vi "Oxford-VRM-Main-Launcher.vi"() -> ()   [LabVIEW 2019]
doc: "This VI will launch the PPMS 2 Instrument backend that will contunously monitor the state of the instrument and log to the DSC. The user has the option of launching a user interface (default) or allowing the backend to run headless. Run \"Launch PPMS2 UI.vi\" here or on a different computer to have a remote user interface. You can also use the APIs like \"Get Temperturature\" interact programmatically with the PPMS 2 Instrument backend."
uses:
  <vilib>/JKI/JKI SMO/SMO/Typedefs/SMOState --Enum.ctl
  SMOs/Instrument.OxfordVRM UI/Instrument.OxfordVRM UI.lvclass
  C:/Program Files (x86)/National Instruments/LabVIEW 2019/vi.lib/JKI/JKI SMO/SMO/SMO.lvclass
  C:/Program Files (x86)/National Instruments/LabVIEW 2019/vi.lib/JKI/JKI SMO/SMO.UI/SMO.UI.lvclass
  C:/Program Files (x86)/National Instruments/LabVIEW 2019/user.lib/LevyLab/Instrument Framework/SMOs/Instrument UI/Instrument UI.lvclass
  SMOs/Instrument.OxfordVRM/Instrument.OxfordVRM.lvclass
  C:/Program Files (x86)/National Instruments/LabVIEW 2019/user.lib/LevyLab/Instrument Framework/SMOs/Instrument/Instrument.lvclass
  <vilib>/JKI/JKI SMO/SMO/SMO.lvclass/SMO.ctl
  <vilib>/JKI/JKI SMO/SMO.UI/SMO.UI.lvclass/SMO.UI.ctl
  <vilib>/JKI/JKI SMO/SMO/Private/ReftoDVR--SMO.vi
  <vilib>/JKI/JKI SMO/SMO.UI/SMO.UI.ReftoDVR.vi
  <vilib>/JKI/JKI SMO/SMO/SMO.lvclass
  <vilib>/JKI/JKI SMO/SMO.UI/SMO.UI.lvclass
  <userlib>/LevyLab/Instrument Framework/SMOs/Instrument UI/Instrument UI.lvclass
  <userlib>/LevyLab/Instrument Framework/SMOs/Instrument/Instrument.lvclass
panel:
  out "version":string="v20/10/28"
  in  "Examine Configuration.ini":bool
  in  "Debug Mode":bool
  in  "Stop Application":bool caption="Stop"
  in  "Start Application":bool caption="Play"
  in  "Splash Status":string="Push Start to Start..." caption="String"
  out "UI SMO State":T1=enum."Stopped"
  out "SMO State":T1
  out "error out":errorcluster
  # "OI 1820"
  # "v"
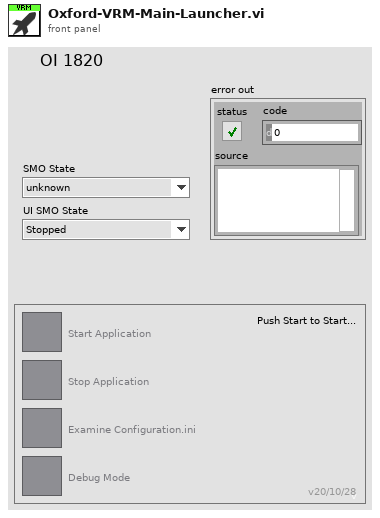
[diagram p1: front panel]
types:
  T1 = typedef "SMO.lvclass/SMOState --Enum.ctl" = enum16{"unknown", "Created", "Started", "Stopped"}
  T2 = enum32{"Invalid", "Standard", "Closed", "Hidden", "Minimized", "Maximized"}
  T3 = enum32{"invalid app kind", "Development System", "Run Time System", "Student Edition", "Embedded LabVIEW", "Evaluation", "Custom"}
  T4 = cluster{"Core":cluster{"Current VI Reference":refnum<vi>, "Close Panel on Exit?":bool}, "Instrument.OxfordVRM":refnum<class "Instrument.OxfordVRM.lvclass">, "Instrument.OxfordVRM UI":refnum<class "Instrument.OxfordVRM UI.lvclass">}
  T5 = cluster{"Current VI Reference":refnum<vi>, "Close Panel on Exit?":bool}
  T6 = typedef "SMO.lvclass/Public Events.ctl" = cluster{"Error":refnum<user-event>, "State":refnum<user-event>, "Reserve State":refnum<user-event>}
  T7 = typedef "SMO.UI.lvclass/PublicEvents--Cluster.ctl" = cluster{"UI Hidden":refnum<user-event>, "UI State":refnum<user-event>}
  T8 = cluster{"Event Registration Refnum":refnum<event-registration>, "Event Registration Refnum":refnum<event-registration>}
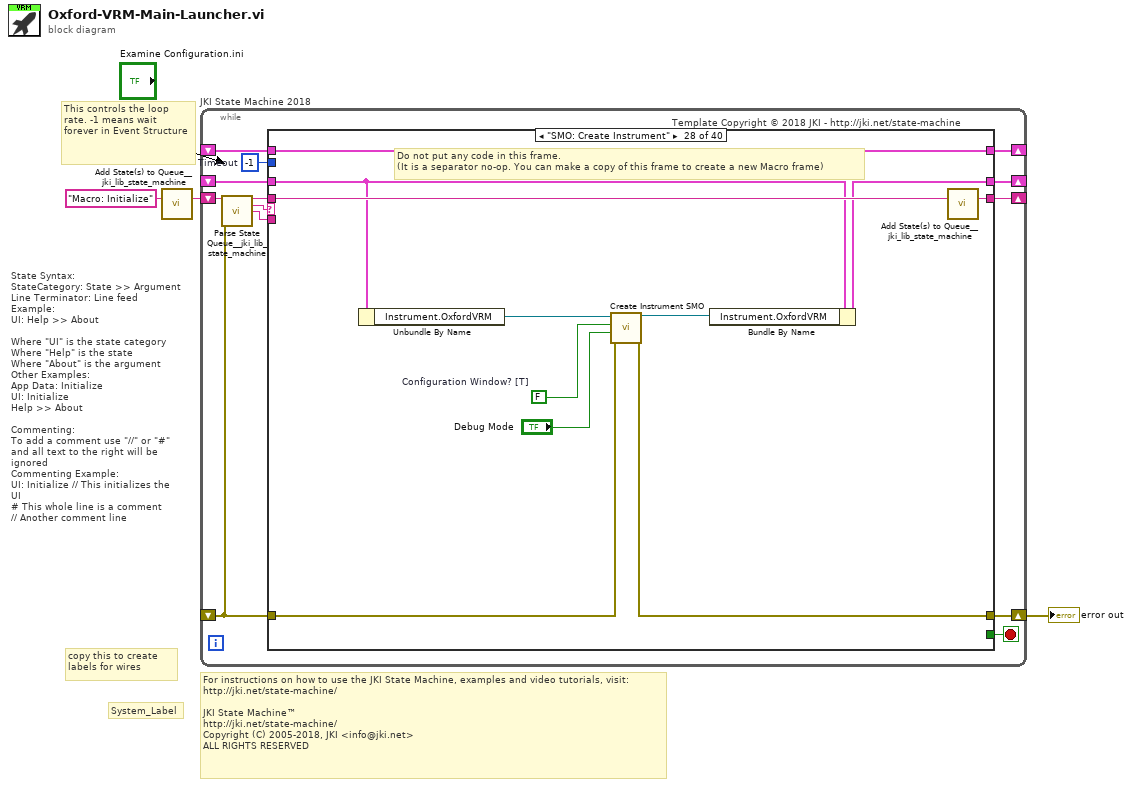
[diagram p0: block diagram]
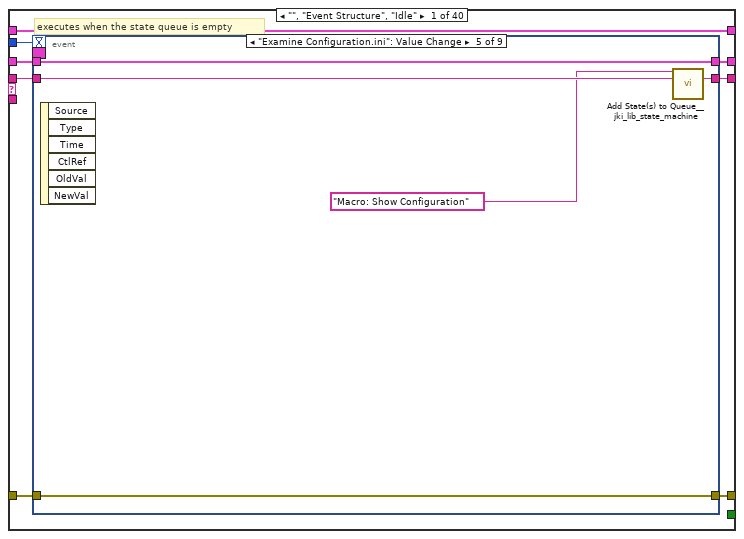
[diagram p2: hidden frame]
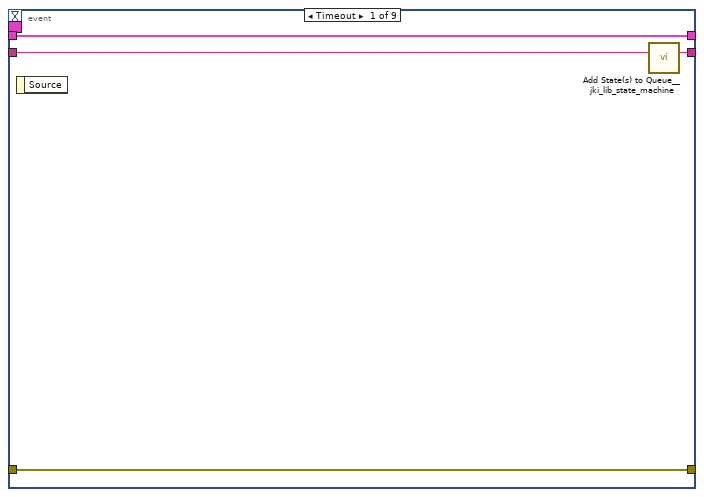
[diagram p3: hidden frame]
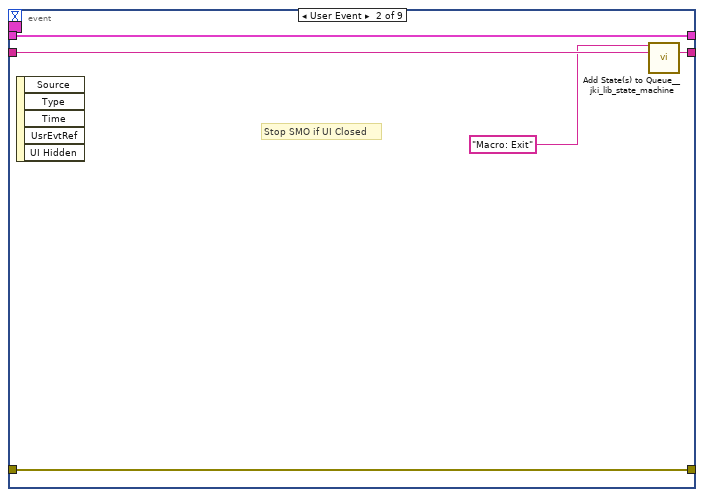
[diagram p4: hidden frame]
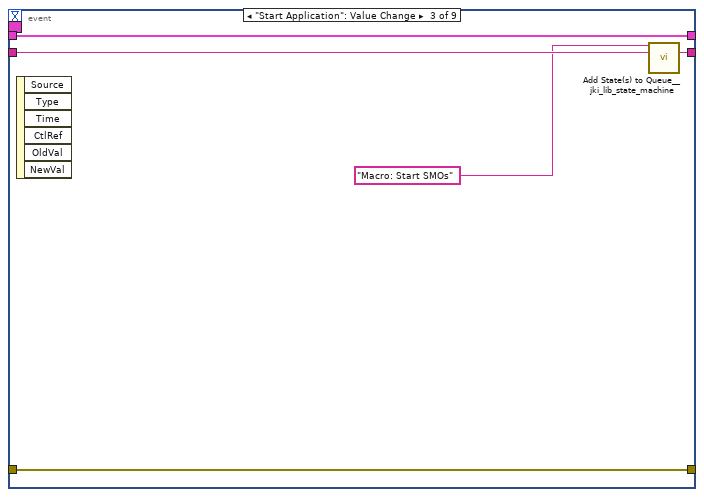
[diagram p5: hidden frame]
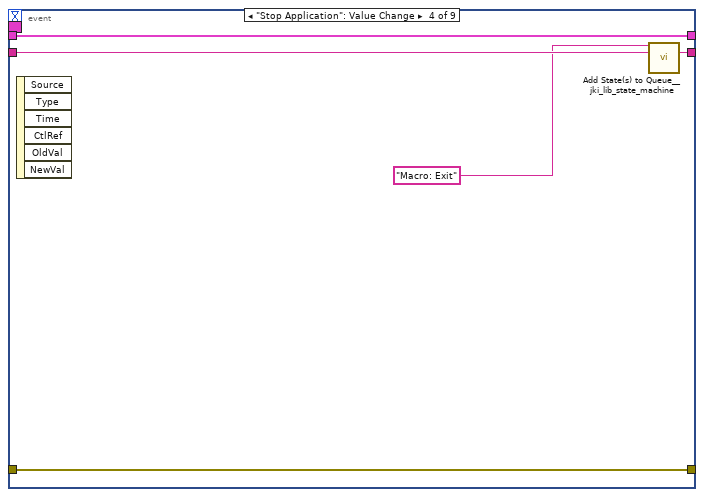
[diagram p6: hidden frame]
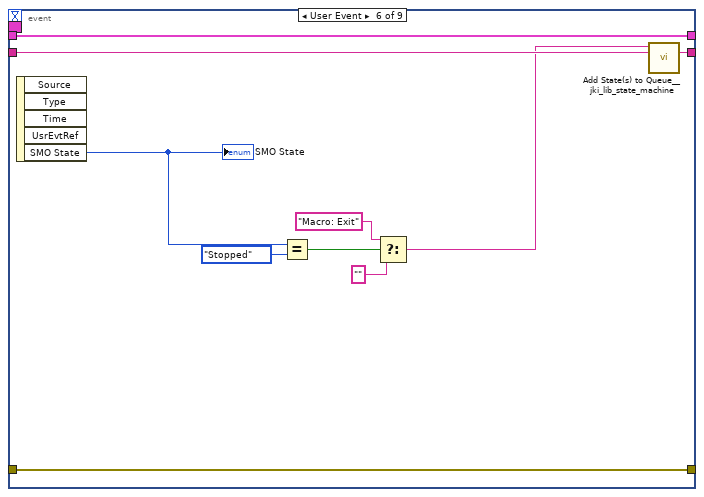
[diagram p7: hidden frame]
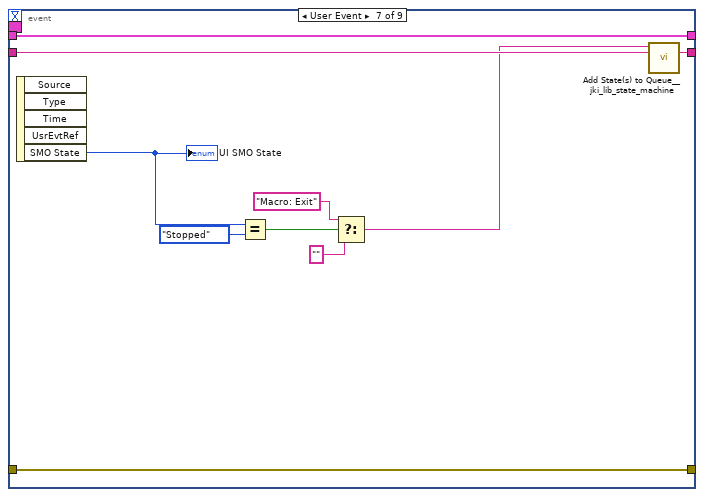
[diagram p8: hidden frame]
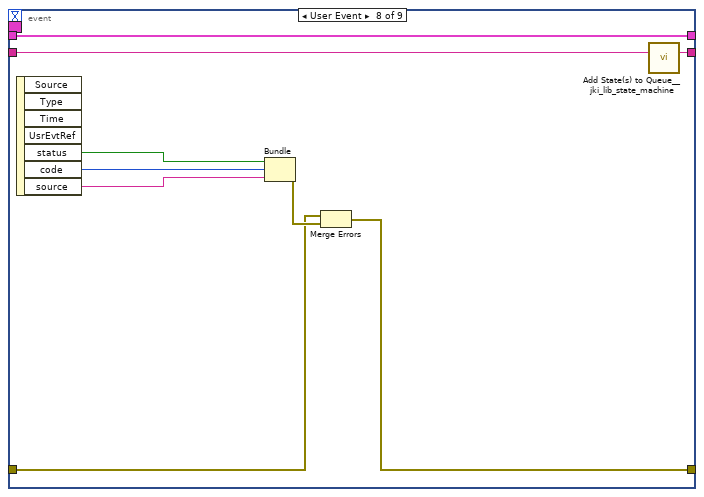
[diagram p9: hidden frame]
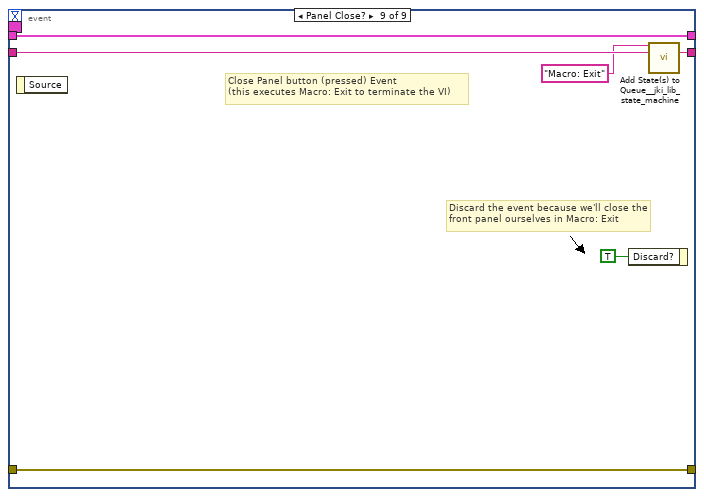
[diagram p10: hidden frame]
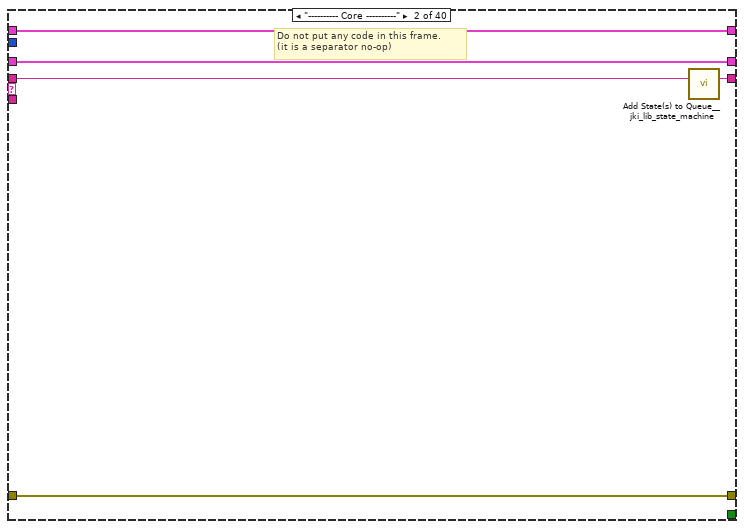
[diagram p11: hidden frame]
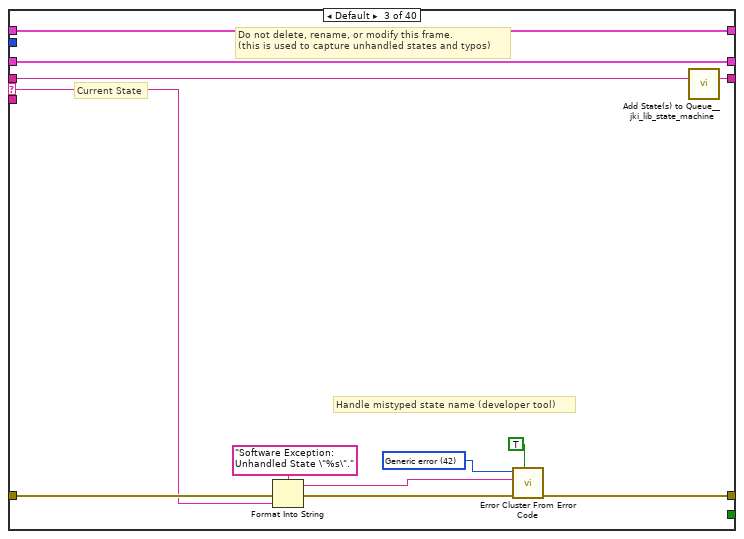
[diagram p12: hidden frame]
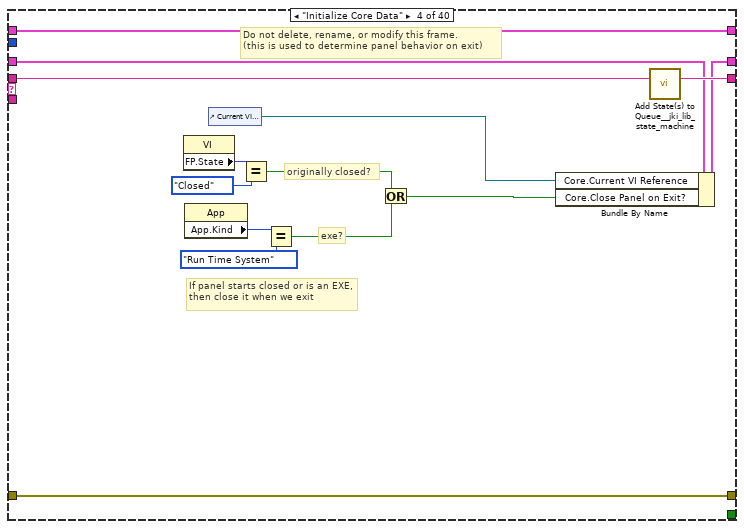
[diagram p13: hidden frame]
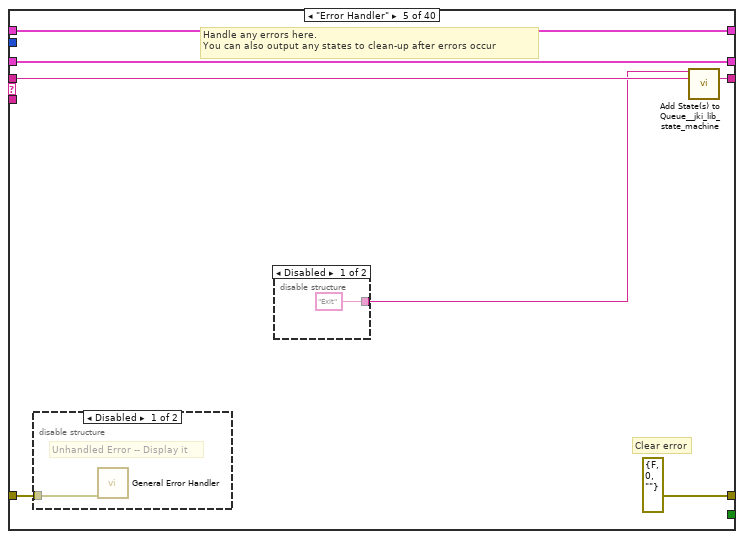
[diagram p14: hidden frame]
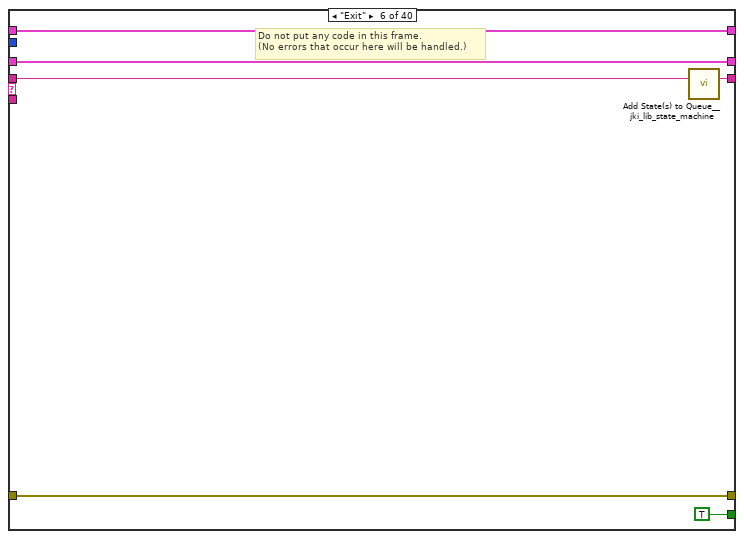
[diagram p17: hidden frame]
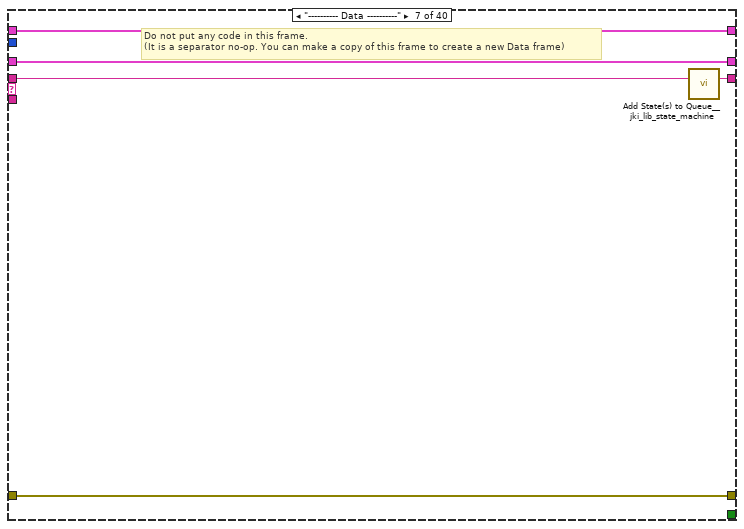
[diagram p18: hidden frame]
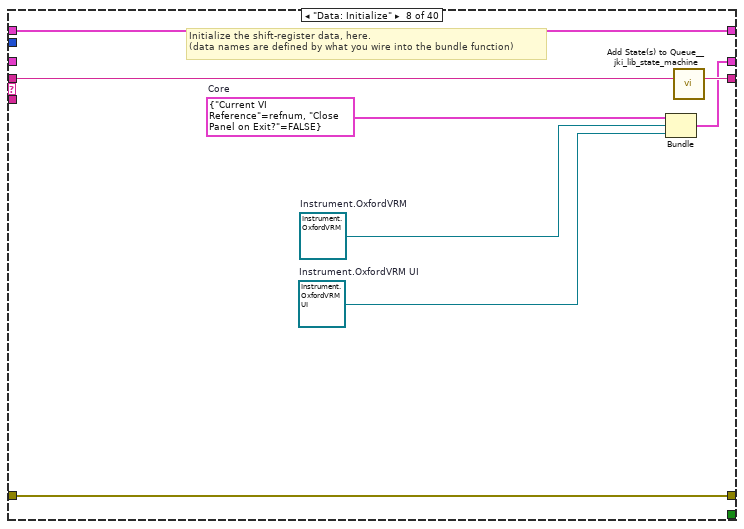
[diagram p19: hidden frame]
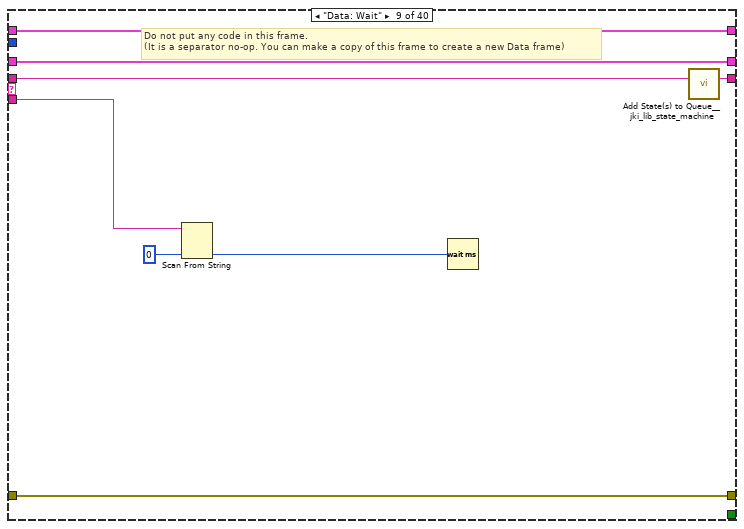
[diagram p20: hidden frame]
diagram:
  # "For instructions on how to use the JKI State Machine, examples and video tutorials, visit:\nhttp://jki.net/state-machine/\n\nJKI State Machine™\nhttp://jki.net/state-machine/\nCopyright (C) 2005-2018, JKI <info@jki.net>\nALL RIGHTS RESERVED"
  # "State Syntax:\nStateCategory: State >> Argument\nLine Terminator: Line feed\nExample:\nUI: Help >> About\n\nWhere \"UI\" is the state category\nWhere \"Help\" is the state\nWhere \"About\" is the argument\nOther Examples:\nApp Data: Initialize\nUI: Initialize\nHelp >> About\n\nCommenting:\nTo add a comment use \"//\" or \"#\" and all text to the right will be ignored\nCommenting Example:\nUI: Initialize // This initializes the UI\n# This whole line is a comment\n// Another comment line"
  # "copy this to create labels for wires"
  # "This controls the loop rate. -1 means wait forever in Event Structure"
  # "System_Label"
  n1 = call <vilib>:"Add State(s) to Queue__jki_lib_state_machine.vi"("State(s) in (\"\")"="Macro: Initialize") -> ("States Out"=w3:string)  [unwired: 14 in]
  n2 = while "JKI State Machine 2018" {
    shift-right: [w9] -> _
    shift-left: _ -> [w4]
    shift-right: [w12] -> w1
    shift-left: _ -> [w7]
    shift-right: [w11] -> _
    shift-left: w3 -> [w13]
    shift-right: [w6] -> _
    shift-left: _ -> [w5]
    stop <- w10 stop-if-true
    w8 = -1  # Timeout
    # "Template Copyright © 2018 JKI - http://jki.net/state-machine"
    n3 = call <vilib>:"Parse State Queue__jki_lib_state_machine.vi"("State Queue"=w13, "Error In (no error)"=w7) -> ("Remaining States"=w15:string, "Current State"=w16:string, "Arguments"=w14:string)  [unwired: 11 in]
    n4 = case shown="\"SMO: Create Instrument\"" w16 {
      selector: w16 -> [_ _ w90 _ _ _ _ _ _ _ _ _ _ _ _ _ _ _ _ _ _ _ _ _ _ _ _ _ _ _ _ _ _ _ _ _ _ _ _ _]
      tunnel: w15 -> [w24 w88 w94 w114 w121 w129 w134 w142 w150 w157 w162 w178 w184 w189 w198 w205 w217 w295 w304 w309 w314 w320 w326 w332 w338 w350 w355 w366 w375 w386 w401 w415 w422 w433 w448 w463 w478 w487 w494 w499]
      tunnel: w14 -> [_ _ _ _ _ _ _ _ w143 _ _ _ _ _ _ w200 w211 _ _ _ _ _ _ _ _ _ _ _ _ _ _ _ _ _ _ _ _ _ w491 _]
      tunnel: [w21 w86 w96 w111 errorcluster {"status"=FALSE, "code"=0, "source"=""} ("error out") w126 w132 w139 w148 w153 w160 w163 w179 w187 w193 w201 w214 w285 w300 w307 w312 w318 w324 w330 w336 w348 w353 w356 w368 w382 w397 w407 w416 w429 w444 w460 w475 w485 w489 w497] -> w12
      tunnel: w7 -> [w20 w86 w95 w111 w117 w126 w132 w139 w148 w154 w160 w169 w180 w187 w195 w202 w215 w286 w299 w307 w312 w318 w324 w330 w336 w348 w353 w357 w369 w378 w393 w408 w417 w426 w441 w458 w471 w485 w490 w497]
      tunnel: [w23 w87 w93 w113 w120 w128 w133 w141 w149 w156 w161 w177 w183 w188 w197 w204 w216 w294 w303 w308 w313 w319 w325 w331 w337 w349 w354 w365 w374 w385 w400 w414 w421 w432 w447 w462 w477 w486 w493 w498] -> w11
      tunnel: [_ _ _ _ _ TRUE _ _ _ _ _ _ _ _ _ _ _ _ _ _ _ _ _ _ _ _ _ _ _ _ _ _ _ _ _ _ _ _ _ _] -> w10
      tunnel: [w19 w85 w92 w112 w118 w127 w131 w140 w147 w152 w159 w172 w182 w186 w196 w203 w213 w283 w298 w306 w311 w317 w323 w329 w335 w347 w352 w363 w370 w383 w398 w411 w419 w430 w445 w459 w474 w484 w492 w496] -> w9
      tunnel: w8 -> [w18 _ _ _ _ _ _ _ _ _ _ _ _ _ _ _ _ _ _ _ _ _ _ _ _ _ _ _ _ _ _ _ _ _ _ _ _ _ _ _]
      tunnel: [w17 w84 w89 w101 w115 w124 w130 w137 w146 w151 w158 w175 w181 w185 w194 w199 w210 w284 w302 w305 w310 w315 w322 w328 w334 w341 w351 w364 w373 w384 w399 w413 w420 w431 w446 w461 w476 w483 w488 w495] -> w6
      tunnel: w5 -> [w17 w84 w89 w101 w115 w124 w130 w137 w146 w151 w158 _ w181 w185 w194 w199 w210 w284 w302 w305 w310 w315 w322 w328 w334 w341 w351 w364 w373 w384 w399 w413 w420 w431 w446 w461 w476 w483 w488 w495]
      tunnel: w4 -> [w22 w85 w92 w107 w118 w127 w131 _ w147 w152 w159 w172 w182 w186 w196 w203 w213 w283 w297 w306 w311 w317 w323 w329 w335 w347 w352 w362 w371 w383 w398 w412 w419 w430 w445 w459 w474 w484 w492 w496]
      frame "", "Event Structure", "Idle" {
        # "executes when the state queue is empty"
        n5 = event shown="[4] \"Examine Configuration.ini\": Value Change" {
          selector: w17 -> [_ _ _ _ _ _ _ _ _]
          dyn-events: _ -> [_ _ _ _ _ _ _ _ _]
          timeout: w18 -> [_ _ _ _ _ _ _ _ _]
          tunnel: w24 -> [w28 w33 w38 w43 w48 w58 w68 w77 w83]
          tunnel: [w27 w32 w37 w42 w47 w57 w67 w76 w82] -> w23
          tunnel: w22 -> [w25 w30 w35 w40 w45 w55 w65 w75 w80]
          tunnel: [w26 w31 w36 w41 w46 w56 w66 w72 w81] -> w21
          tunnel: w20 -> [w26 w31 w36 w41 w46 w56 w66 w73 w81]
          tunnel: [w25 w30 w35 w40 w45 w55 w65 w75 w80] -> w19
          event Timeout {
            n6 = event-data() -> ()  [unwired: 1 in, 1 out]
            n7 = call <vilib>:"Add State(s) to Queue__jki_lib_state_machine.vi"("State(s) in (\"\")"=w28) -> ("States Out"=w27:string)  [unwired: 14 in]
          }
          event User Event {
            # "Stop SMO if UI Closed"
            n8 = event-data() -> ()  [unwired: 1 in, 5 out]
            n9 = call <vilib>:"Add State(s) to Queue__jki_lib_state_machine.vi"("State(s) in Front (\"\")"="Macro: Exit" ("State(s) in Front (\"\")"), "State(s) in (\"\")"=w33) -> ("States Out"=w32:string)  [unwired: 13 in]
          }
          event "Start Application": Value Change {
            n10 = event-data() -> ()  [unwired: 1 in, 6 out]
            n11 = call <vilib>:"Add State(s) to Queue__jki_lib_state_machine.vi"("State(s) in Front (\"\")"="Macro: Start SMOs" ("State(s) in Front (\"\")"), "State(s) in (\"\")"=w38) -> ("States Out"=w37:string)  [unwired: 13 in]
          }
          event "Stop Application": Value Change {
            n12 = event-data() -> ()  [unwired: 1 in, 6 out]
            n13 = call <vilib>:"Add State(s) to Queue__jki_lib_state_machine.vi"("State(s) in Front (\"\")"="Macro: Exit" ("State(s) in Front (\"\")"), "State(s) in (\"\")"=w43) -> ("States Out"=w42:string)  [unwired: 13 in]
          }
          event "Examine Configuration.ini": Value Change {
            n14 = event-data() -> ()  [unwired: 1 in, 6 out]
            n15 = call <vilib>:"Add State(s) to Queue__jki_lib_state_machine.vi"("State(s) in Front (\"\")"="Macro: Show Configuration" ("State(s) in Front (\"\")"), "State(s) in (\"\")"=w48) -> ("States Out"=w47:string)  [unwired: 13 in]
          }
          event User Event {
            n16 = event-data() -> ("SMO State"=w50:T1)  [unwired: 1 in, 4 out]
            "SMO State" <- w50
            n17 = Equal?(x=w50, y=SMOState_--Enum."Stopped") -> (x = y?=w53:bool)
            n18 = Select(t="Macro: Exit", s=w53, f="" ("State(s) in Front (\"\")")) -> (s? t:f=w49:string)
            n19 = call <vilib>:"Add State(s) to Queue__jki_lib_state_machine.vi"("State(s) in Front (\"\")"=w49, "State(s) in (\"\")"=w58) -> ("States Out"=w57:string)  [unwired: 13 in]
          }
          event User Event {
            n20 = event-data() -> ("SMO State"=w59:T1)  [unwired: 1 in, 4 out]
            "UI SMO State" <- w59
            n21 = Equal?(x=w59, y=SMOState_--Enum."Stopped") -> (x = y?=w63:bool)
            n22 = Select(t="Macro: Exit", s=w63, f="" ("State(s) in Front (\"\")")) -> (s? t:f=w61:string)
            n23 = call <vilib>:"Add State(s) to Queue__jki_lib_state_machine.vi"("State(s) in Front (\"\")"=w61, "State(s) in (\"\")"=w68) -> ("States Out"=w67:string)  [unwired: 13 in]
          }
          event User Event {
            n24 = event-data() -> ("status"=w69:bool, "code"=w71:i32, "source"=w70:string)  [unwired: 1 in, 4 out]
            n25 = Bundle("status"=w69, "code"=w71, "source"=w70) -> (w74:errorcluster)  [unwired: 1 in]
            n26 = Merge Errors(w73, w74) -> (w72:errorcluster)
            n27 = call <vilib>:"Add State(s) to Queue__jki_lib_state_machine.vi"("State(s) in (\"\")"=w77) -> ("States Out"=w76:string)  [unwired: 14 in]
          }
          event Panel Close? {
            # "Discard the event because we'll close the front panel ourselves in Macro: Exit"
            # "Close Panel button (pressed) Event\n(this executes Macro: Exit to terminate the VI)"
            n28 = event-data() -> ()  [unwired: 1 in, 1 out]
            n29 = event-data("Discard?"=TRUE) -> ()  [unwired: 1 in, 1 out]
            n30 = call <vilib>:"Add State(s) to Queue__jki_lib_state_machine.vi"("State(s) in Front (\"\")"="Macro: Exit", "State(s) in (\"\")"=w83) -> ("States Out"=w82:string)  [unwired: 13 in]
          }
        }
      }
      frame "---------- Core ----------" {
        # "Do not put any code in this frame.\n(it is a separator no-op)"
        n31 = call <vilib>:"Add State(s) to Queue__jki_lib_state_machine.vi"("State(s) in (\"\")"=w88) -> ("States Out"=w87:string)  [unwired: 14 in]
      }
      frame Default {
        w99 = 42 items=["No error", "Argument error", "Memory is full", "Out of zone", "End of file", "File already open", "Generic file I/O error", "File not found", "File permission error", "Disk is full", "Duplicate path", "Too many files open", "System feature not enabled", "Resource file not found", "Cannot add resource", "Resource not found", "Image not found", "Image memory error", "Pen does not exist", "Config type invalid", "Config token not found", "Config parse error", "Config memory error", "Bad external code format", "Bad external code offset", "External code not present", "Null window", "Destroy window error", "Null menu", "Print aborted", "Bad print record", "Print driver error", "Windows error during printing", "Memory error during printing", "Print dialog error", "Generic print error", "Invalid device refnum", "Device not found", "Device parameter error", "Device unit error", "Cannot open device", "Device call aborted", "Generic error", "Cancelled by user", "Object ID too low", "Object ID too high", "Object not in heap", "Unknown heap", "Unknown object (invalid DefProc)", "Unknown object (DefProc not in table)", "Message out of range", "Invalid (null) method", "Unknown message", "Manager call not supported", "Bad address", "Network operation in progress", "Network operation timed out", "Connection is busy", "Network attribute not supported", "Network error", "Address in use", "System out of memory", "Connection aborted", "Connection refused", "Not connected", "Already connected", "Connection closed", "Initialization error (interapplication manager)", "Bad occurrence", "Wait on unbound occurrence handler", "Occurrence queue overflow", "Datalog type conflict", "Unused", "Unrecognized type (interapplication manager)", "Memory corrupt", "Failed to make temporary DLL", "Old CIN version", "Drag socket not found", "Failed to load drop-object", "Failed to register OLE object", "Failed to release OLE object", "Format specifier type mismatch", "Unknown format specifier", "Too few format specifiers", "Too many format specifiers", "Scan failed", "Newer CIN version", "Error converting to variant", "Runtime menu error", "Password tampered", "Variant attribute not found", "Incompatible variant data type", "Event data is not available", "Event Store is not present", "Occurrence is not found", "Event Queue is not created", "Event info is not available", "Refnum passed is NULL", "Error retrieving Class GUID", "Error retrieving CoClass GUID", "Error retrieving TypeLib GUID.", "Bad built application magic bytes.", "Specific driver is different from the specific driver associated with the Logical Name.", "There is no session opened to the class driver.", "Max Error", "MAX - Error with config objects", "MAX - Error loading configuration", "MAX - Group not supported"]
        # "Current State"
        # "Do not delete, rename, or modify this frame.\n(this is used to capture unhandled states and typos)"
        # "Handle mistyped state name (developer tool)"
        n32 = Format Into String(format string="Software Exception: Unhandled State \"%s\"." ("message"), error in=w95, w90) -> (resulting string=w98:string, error out=w97:errorcluster)  [unwired: 1 in]
        n33 = call <vilib>:"Error Cluster From Error Code.vi"("show call chain? (False)"=TRUE, "error in (no error)"=w97, "error message (\"\")"=w98, "error code (0)"=w99) -> ("error out"=w96:errorcluster)  [unwired: 5 in]
        n34 = call <vilib>:"Add State(s) to Queue__jki_lib_state_machine.vi"("State(s) in (\"\")"=w94) -> ("States Out"=w93:string)  [unwired: 14 in]
      }
      frame "Initialize Core Data" {
        # "Do not delete, rename, or modify this frame.\n(this is used to determine panel behavior on exit)"
        # "originally closed?"
        # "exe?"
        # "If panel starts closed or is an EXE, then close it when we exit"
        n35 = property class="VI"() -> ("FP.State"=w104:T2)  [unwired: 2 in, 2 out]
        n36 = property class="App"() -> ("App.Kind"=w110:T3)  [unwired: 2 in, 2 out]
        n37 = control-ref of="Current VI Reference"() -> (w105:refnum<vi>)
        n38 = Equal?(x=w104, y=T2."Closed" ("Front Panel Window:State")) -> (x = y?=w102:bool)
        n39 = Equal?(x=w110, y=T3."Run Time System" ("Application:Kind")) -> (x = y?=w108:bool)
        n40 = Or(x=w102, y=w108) -> (x .or. y?=w106:bool)
        n41 = Bundle By Name(cluster=w107, "Core.Current VI Reference"=w105, "Core.Close Panel on Exit?"=w106) -> (w112:T4)
        n42 = call <vilib>:"Add State(s) to Queue__jki_lib_state_machine.vi"("State(s) in (\"\")"=w114) -> ("States Out"=w113:string)  [unwired: 14 in]
      }
      frame "Error Handler" {
        # "Handle any errors here.\nYou can also output any states to clean-up after errors occur"
        # "Clear error"
        n43 = disable-structure shown="Disabled" {
          disable-tunnel: w117 -> [w123 _]
          frame Disabled {
            # "Unhandled Error -- Display it"
            n44 = call <vilib>:"General Error Handler.vi"("error in (no error)"=w123) -> ()  [unwired: 10 in, 5 out]
          }
          frame Enabled {
          }
        }
        n45 = disable-structure shown="Disabled" {
          disable-tunnel: ["Exit" _] -> w116
          frame Disabled {
          }
          frame Enabled {
          }
        }
        n46 = call <vilib>:"Add State(s) to Queue__jki_lib_state_machine.vi"("State(s) in Front (\"\")"=w116, "State(s) in (\"\")"=w121) -> ("States Out"=w120:string)  [unwired: 13 in]
      }
      frame "Exit" {
        # "Do not put any code in this frame.\n(No errors that occur here will be handled.)"
        n47 = call <vilib>:"Add State(s) to Queue__jki_lib_state_machine.vi"("State(s) in (\"\")"=w129) -> ("States Out"=w128:string)  [unwired: 14 in]
      }
      frame "---------- Data ----------" {
        # "Do not put any code in this frame.\n(It is a separator no-op. You can make a copy of this frame to create a new Data frame)"
        n48 = call <vilib>:"Add State(s) to Queue__jki_lib_state_machine.vi"("State(s) in (\"\")"=w134) -> ("States Out"=w133:string)  [unwired: 14 in]
      }
      frame "Data: Initialize" {
        w136 = refnum<class "Instrument.OxfordVRM.lvclass"> refnum  # Instrument.OxfordVRM
        w135 = refnum<class "Instrument.OxfordVRM UI.lvclass"> refnum  # Instrument.OxfordVRM UI
        w138 = T5 {"Current VI Reference"=refnum, "Close Panel on Exit?"=FALSE}  # Core
        # "Initialize the shift-register data, here.\n(data names are defined by what you wire into the bundle function)"
        n49 = Bundle("Core"=w138, "Instrument.OxfordVRM"=w136, "Instrument.OxfordVRM UI"=w135) -> (w140:T4)  [unwired: 1 in]
        n50 = call <vilib>:"Add State(s) to Queue__jki_lib_state_machine.vi"("State(s) in (\"\")"=w142) -> ("States Out"=w141:string)  [unwired: 14 in]
      }
      frame "Data: Wait" {
        # "Do not put any code in this frame.\n(It is a separator no-op. You can make a copy of this frame to create a new Data frame)"
        n51 = Scan From String(input string=w143, default 1=u32 0) -> (output 1=w144:u32)  [unwired: 3 in, 3 out]
        n52 = Wait (ms)(milliseconds to wait=w144) -> ()  [unwired: 1 out]
        n53 = call <vilib>:"Add State(s) to Queue__jki_lib_state_machine.vi"("State(s) in (\"\")"=w150) -> ("States Out"=w149:string)  [unwired: 14 in]
      }
      frame "Data: Cleanup" {
        # "Cleanup any data and references, here.\n(this is called automatically, by the Macro: Exit)"
        n54 = Unbundle By Name(w152) -> ("Core.Current VI Reference"=w155:refnum<vi>)
        n55 = Close Reference(reference=w155, error in (no error)=w154) -> (error out=w153:errorcluster)
        n56 = call <vilib>:"Add State(s) to Queue__jki_lib_state_machine.vi"("State(s) in (\"\")"=w157) -> ("States Out"=w156:string)  [unwired: 14 in]
      }
      frame "---------- Events ----------" {
        # "Do not put any code in this frame.\n(It is a separator no-op. You can make a copy of this frame to create a new UI frame)"
        n57 = call <vilib>:"Add State(s) to Queue__jki_lib_state_machine.vi"("State(s) in (\"\")"=w162) -> ("States Out"=w161:string)  [unwired: 14 in]
      }
      frame "Events: Register" {
        # "Do not put any code in this frame.\n(It is a separator no-op. You can make a copy of this frame to create a new UI frame)"
        n58 = Unbundle By Name(w172) -> ("Instrument.OxfordVRM"=w171:refnum<class "Instrument.OxfordVRM.lvclass">, "Instrument.OxfordVRM UI"=w170:refnum<class "Instrument.OxfordVRM UI.lvclass">)
        n59 = call <vilib>:"GetPublicEvents.vi"("error in (no error)"=w169, "SMO"=w171) -> ("error out"=w168:errorcluster, "Public Events"=w173:T6)  [unwired: 7 in, 1 out]
        n60 = call <vilib>:"GetPublicEvents.vi"("error in (no error)"=w168, "SMO"=w170) -> ("error out"=w164:errorcluster, "Public Events"=w174:T6, "SMO out"=w166:refnum<class "Instrument.OxfordVRM UI.lvclass">)  [unwired: 7 in]
        n61 = register-events(w173) -> (reference out=w176:refnum<event-registration>)  [unwired: 2 in, 1 out]
        n62 = call <vilib>:"SMO.UI.GetPublicEvents.vi"("error in (no error)"=w164, "SMO.UI"=w166) -> ("error out"=w163:errorcluster, "SMO.UI Public Events"=w165:T7)  [unwired: 7 in, 1 out]
        n63 = register-events(w174, w165) -> (reference out=w167:refnum<event-registration>)  [unwired: 2 in, 1 out]
        n64 = Bundle("Event Registration Refnum"=w176, "Event Registration Refnum"=w167) -> (w175:T8)  [unwired: 1 in]
        n65 = call <vilib>:"Add State(s) to Queue__jki_lib_state_machine.vi"("State(s) in (\"\")"=w178) -> ("States Out"=w177:string)  [unwired: 14 in]
      }
      frame "Events: Unregister" {
        # "Do not put any code in this frame.\n(It is a separator no-op. You can make a copy of this frame to create a new UI frame)"
        n66 = Unregister For Events(event registration refnum=w181, error in=w180) -> (error out=w179:errorcluster)
        n67 = call <vilib>:"Add State(s) to Queue__jki_lib_state_machine.vi"("State(s) in (\"\")"=w184) -> ("States Out"=w183:string)  [unwired: 14 in]
      }
      frame "---------- UI ----------" {
        # "Do not put any code in this frame.\n(It is a separator no-op. You can make a copy of this frame to create a new UI frame)"
        n68 = call <vilib>:"Add State(s) to Queue__jki_lib_state_machine.vi"("State(s) in (\"\")"=w189) -> ("States Out"=w188:string)  [unwired: 14 in]
      }
      frame "UI: Initialize" {
        # "Initialize the User Interface, here.\n(this is called automatically, by the Macro: Init)"
        n69 = invoke on="Stop Application" class="Bool" method="Reinit To Default"() -> ()  [unwired: 3 in, 3 out]
        n70 = invoke on="error out" class="Clust (strict)" method="Reinit To Default"() -> ()  [unwired: 3 in, 3 out]
        n71 = invoke on="SMO State" class="Enum (strict)" method="Reinit To Default"() -> ()  [unwired: 3 in, 3 out]
        n72 = invoke on="Start Application" class="Bool" method="Reinit To Default"() -> ()  [unwired: 3 in, 3 out]
        n73 = call <userlib>:"Fit VI window to Largest Dec__ogtk.vi"("error in (no error)"=w195) -> ("error out"=w193:errorcluster)  [unwired: 5 in, 1 out]
        n74 = call <userlib>:"MGI Get Executable Version.vi"() -> ("Version"=w192:string)  [unwired: 7 in]
        n75 = Format Into String(format string="v%s" ("version"), w192) -> (resulting string=→"version":string)  [unwired: 2 in, 1 out]
        n76 = call <vilib>:"Add State(s) to Queue__jki_lib_state_machine.vi"("State(s) in (\"\")"=w198) -> ("States Out"=w197:string)  [unwired: 14 in]
      }
      frame "UI: Cursor Set" {
        # "Argument"
        # "Set and Unset Cursor Busy.\n(Usage: \"UI: Cursor Set >> Busy|Idle\")"
        n77 = case shown="\"Idle\", Default" w200 {
          tunnel: w202 -> [w207 w209]
          tunnel: [w206 w208] -> w201
          frame "Idle", Default {
            n78 = call <vilib>:"Unset Busy.vi"("error in (no error)"=w207) -> ("error out"=w206:errorcluster)  [unwired: 10 in]
          }
          frame "Busy" {
            n79 = call <vilib>:"Set Busy.vi"("error in (no error)"=w209) -> ("error out"=w208:errorcluster)  [unwired: 9 in, 1 out]
          }
        }
        n80 = call <vilib>:"Add State(s) to Queue__jki_lib_state_machine.vi"("State(s) in (\"\")"=w205) -> ("States Out"=w204:string)  [unwired: 14 in]
      }
      frame "UI: Front Panel State" {
        # "Argument"
        # "Set Front Panel Open or Closed\n(Usage: \"UI: Front Panel State >> Open|Close\")"
        n81 = Unbundle By Name(w213) -> ("Core.Current VI Reference"=w212:refnum<vi>)
        n82 = case shown="\"Open\", \"Standard\", Default" w211 {
          tunnel: w215 -> [w223 w238 w249 w262 w275]
          tunnel: [w225 w239 w251 w264 w277] -> w214
          tunnel: w212 -> [w224 w236 w250 w263 w276]
          frame "Open", "Standard", Default {
            w218 = T2."Standard" ("State")
            n83 = property class="VI"(reference=w224, error in=w223) -> (reference out=w221:refnum<vi>, error out=w222:errorcluster, "FP.State"=w220:T2)
            n84 = Not Equal?(x=w220, y=w218) -> (x != y?=w219:bool)
            n85 = case shown="False" w219 {
              tunnel: [w229 w231] -> w225
              tunnel: w222 -> [w228 w231]
              tunnel: w221 -> [w227 _]
              tunnel: w218 -> [w226 _]
              frame True {
                n86 = invoke class="VI" method="FP.Open"(reference=w227, error in=w228, "Activate"=TRUE, "State"=w226) -> (error out=w229:errorcluster)  [unwired: 1 in, 4 out]
              }
              frame False {
              }
            }
          }
          frame "Close", "Closed" {
            n87 = property class="VI"(reference=w236, error in=w238) -> (reference out=w235:refnum<vi>, error out=w237:errorcluster, "FP.State"=w233:T2)
            n88 = Not Equal?(x=w233, y=T2."Closed" ("Front Panel Window:State")) -> (x != y?=w232:bool)
            n89 = case shown="True" w232 {
              tunnel: [w240 w243] -> w239
              tunnel: w237 -> [w240 w242]
              tunnel: w235 -> [_ w241]
              frame False {
              }
              frame True {
                n90 = invoke class="VI" method="FP.Close"(reference=w241, error in=w242) -> (error out=w243:errorcluster)  [unwired: 1 in, 2 out]
              }
            }
          }
          frame "Hidden", "Hide" {
            w244 = T2."Hidden" ("State")
            n91 = property class="VI"(reference=w250, error in=w249) -> (reference out=w247:refnum<vi>, error out=w248:errorcluster, "FP.State"=w246:T2)
            n92 = Not Equal?(x=w246, y=w244) -> (x != y?=w245:bool)
            n93 = case shown="True" w245 {
              tunnel: [w255 w256] -> w251
              tunnel: w248 -> [w254 w256]
              tunnel: w247 -> [w253 _]
              tunnel: w244 -> [w252 _]
              frame True {
                n94 = invoke class="VI" method="FP.Open"(reference=w253, error in=w254, "State"=w252) -> (error out=w255:errorcluster)  [unwired: 2 in, 4 out]
              }
              frame False {
              }
            }
          }
          frame "Minimize", "Minimized" {
            w257 = T2."Minimized" ("State")
            n95 = property class="VI"(reference=w263, error in=w262) -> (reference out=w260:refnum<vi>, error out=w261:errorcluster, "FP.State"=w259:T2)
            n96 = Not Equal?(x=w259, y=w257) -> (x != y?=w258:bool)
            n97 = case shown="True" w258 {
              tunnel: [w268 w269] -> w264
              tunnel: w261 -> [w267 w269]
              tunnel: w260 -> [w266 _]
              tunnel: w257 -> [w265 _]
              frame True {
                n98 = invoke class="VI" method="FP.Open"(reference=w266, error in=w267, "State"=w265) -> (error out=w268:errorcluster)  [unwired: 2 in, 4 out]
              }
              frame False {
              }
            }
          }
          frame "Maximize", "Maximized" {
            w270 = T2."Maximized" ("State")
            n99 = property class="VI"(reference=w276, error in=w275) -> (reference out=w273:refnum<vi>, error out=w274:errorcluster, "FP.State"=w272:T2)
            n100 = Not Equal?(x=w272, y=w270) -> (x != y?=w271:bool)
            n101 = case shown="True" w271 {
              tunnel: [w281 w282] -> w277
              tunnel: w274 -> [w280 w282]
              tunnel: w273 -> [w279 _]
              tunnel: w270 -> [w278 _]
              frame True {
                n102 = invoke class="VI" method="FP.Open"(reference=w279, error in=w280, "State"=w278) -> (error out=w281:errorcluster)  [unwired: 2 in, 4 out]
              }
              frame False {
              }
            }
          }
        }
        n103 = call <vilib>:"Add State(s) to Queue__jki_lib_state_machine.vi"("State(s) in (\"\")"=w217) -> ("States Out"=w216:string)  [unwired: 14 in]
      }
      frame "UI: Set Background Color" {
        # "Do not put any code in this frame.\n(It is a separator no-op. You can make a copy of this frame to create a new UI frame)"
        n104 = property class="VI"(error in=w286) -> (error out=w288:errorcluster, "Panel"=w289:refnum<vi>)  [unwired: 1 in, 1 out]
        n105 = property class="Pnl"(reference=w289, error in=w288) -> (error out=w287:errorcluster, "Panes[]"=w290:refnum<vi>[])  [unwired: 1 out]
        n106 = Index Array(array=w290, index=0) -> (element=w292:refnum<vi>)
        n107 = property class="Pane"(reference=w292, error in=w287, "PaneColor"=u32 16777238 ("Color Box")) -> (error out=w285:errorcluster)  [unwired: 1 out]
        n108 = call <vilib>:"Add State(s) to Queue__jki_lib_state_machine.vi"("State(s) in (\"\")"=w295) -> ("States Out"=w294:string)  [unwired: 14 in]
      }
      frame "UI: Open Configuration.ini" {
        # "Do not put any code in this frame.\n(It is a separator no-op. You can make a copy of this frame to create a new UI frame)"
        n109 = Unbundle By Name(w297) -> ("Instrument.OxfordVRM"=w301:refnum<class "Instrument.OxfordVRM.lvclass">)
        n110 = call <userlib>:"Examine Configuration.vi"("error in (no error)"=w299, "Instrument in"=w301) -> ("error out"=w300:errorcluster, "Instrument out"=w296:refnum<class "Instrument.OxfordVRM.lvclass">)  [unwired: 8 in]
        n111 = Bundle By Name(cluster=w297, "Instrument.OxfordVRM"=w296) -> (w298:T4)
        n112 = call <vilib>:"Add State(s) to Queue__jki_lib_state_machine.vi"("State(s) in (\"\")"=w304) -> ("States Out"=w303:string)  [unwired: 14 in]
      }
      frame "UI: Exit" {
        # "Do not put any code in this frame.\n(It is a separator no-op. You can make a copy of this frame to create a new UI frame)"
        n113 = invoke on="Start Application" class="Bool" method="Reinit To Default"() -> ()  [unwired: 3 in, 3 out]
        n114 = invoke on="Stop Application" class="Bool" method="Reinit To Default"() -> ()  [unwired: 3 in, 3 out]
        n115 = call <vilib>:"Add State(s) to Queue__jki_lib_state_machine.vi"("State(s) in (\"\")"=w309) -> ("States Out"=w308:string)  [unwired: 14 in]
      }
      frame "---------- Macro ----------" {
        # "Do not put any code in this frame.\n(It is a separator no-op. You can make a copy of this frame to create a new Macro frame)"
        n116 = call <vilib>:"Add State(s) to Queue__jki_lib_state_machine.vi"("State(s) in (\"\")"=w314) -> ("States Out"=w313:string)  [unwired: 14 in]
      }
      frame "Macro: Initialize" {
        # "Initialization Macro\n(This is called once, when the VI starts)"
        n117 = call <vilib>:"Add State(s) to Queue__jki_lib_state_machine.vi"("State(s) in Front (\"\")"="Data: Initialize\nInitialize Core Data\n//Events: Register\nUI: Initialize\nUI: Front Panel State >> Open\nUI: Set Background Color\nSplash: Set Status >> Push Start to Start...", "State(s) in (\"\")"=w320) -> ("States Out"=w319:string)  [unwired: 13 in]
      }
      frame "Macro: Show Configuration" {
        # "Do not put any code in this frame.\n(It is a separator no-op. You can make a copy of this frame to create a new Macro frame)"
        n118 = call <vilib>:"Add State(s) to Queue__jki_lib_state_machine.vi"("State(s) in Front (\"\")"="Splash: Set Status >> Opening Configuration...\nUI: Open Configuration.ini\nData: Wait >> 1000\nSplash: Set Status >> ...", "State(s) in (\"\")"=w326) -> ("States Out"=w325:string)  [unwired: 13 in]
      }
      frame "Macro: Start SMOs" {
        # "Do not put any code in this frame.\n(It is a separator no-op. You can make a copy of this frame to create a new Macro frame)"
        n119 = call <vilib>:"Add State(s) to Queue__jki_lib_state_machine.vi"("State(s) in Front (\"\")"="Splash: Set Status >> Creating Instrument...\nSMO: Create Instrument\nData: Wait >> 100\nSplash: Set Status >> Creating Instrument UI...\nSMO: Create Instrument UI\nData: Wait >> 100\nSplash: Set Status >> Registering Events...\nEvents: Register\nData: Wait >> 100\nSplash: Set Status >> Starting Instrument...\nSMO: Start Instrument\nData: Wait >> 100\nSplash: Set Status >> Instrument Process Started...\nData: Wait >> 100\nSplash: Set Status >> Starting User Interface...\nSMO: Start Instrument UI\nData: Wait >> 100\nUI: Front Panel State >> Hide\nSMO: Show Instrument UI" ("State(s) in Front (\"\")"), "State(s) in (\"\")"=w332) -> ("States Out"=w331:string)  [unwired: 13 in]
      }
      frame "Macro: Stop SMOs" {
        # "Do not put any code in this frame.\n(It is a separator no-op. You can make a copy of this frame to create a new Macro frame)"
        n120 = call <vilib>:"Add State(s) to Queue__jki_lib_state_machine.vi"("State(s) in Front (\"\")"="UI: Front Panel State >> Show\nSplash: Set Status >> Stopping Instrument...\nSMO: Stop Instrument\nData: Wait >> 100\nSplash: Set Status >> Destroying Instrument...\nSMO: Destroy Instrument\nData: Wait >> 100\nSplash: Set Status >>Hiding UI...\nSMO: Hide Instrument UI\nData: Wait >> 100\nSplash: Set Status >> Stopping UI...\nSMO: Stop Instrument UI\nData: Wait >> 100\nSplash: Set Status >> Destroying UI...\nSMO: Destroy Instrument UI" ("State(s) in Front (\"\")"), "State(s) in (\"\")"=w338) -> ("States Out"=w337:string)  [unwired: 13 in]
      }
      frame "Macro: Exit" {
        # "Exit Macro\n(This is called once, when the VI exits)"
        n121 = Unbundle By Name(w347) -> ("Core.Close Panel on Exit?"=w346:bool)
        n122 = Select(t="UI: Front Panel State >> Open", s=w346, f="") -> (s? t:f=w343:string)
        n123 = call <vilib>:"Add State(s) to Queue__jki_lib_state_machine.vi"("State(s) in Front (\"\")"="UI: Front Panel State >> Close\nMacro: Stop SMOs\nUI: Exit", "State(s) in (\"\")"=w343, "State(s) at Back (\"\")"="Data: Cleanup\nEvents: Unregister\nExit") -> ("States Out"=w342:string)  [unwired: 12 in]
        n124 = call <vilib>:"Add State(s) to Queue__jki_lib_state_machine.vi"("State(s) in Front (\"\")"=w342, "State(s) in (\"\")"=w350) -> ("States Out"=w349:string)  [unwired: 13 in]
      }
      frame "---------- SMO ----------" {
        # "Do not put any code in this frame.\n(It is a separator no-op. You can make a copy of this frame to create a new Macro frame)"
        n125 = call <vilib>:"Add State(s) to Queue__jki_lib_state_machine.vi"("State(s) in (\"\")"=w355) -> ("States Out"=w354:string)  [unwired: 14 in]
      }
      frame "SMO: Create Instrument" {
        w359 = FALSE  # Configuration Window? [T]
        # "Do not put any code in this frame.\n(It is a separator no-op. You can make a copy of this frame to create a new Macro frame)"
        n126 = Unbundle By Name(w362) -> ("Instrument.OxfordVRM"=w361:refnum<class "Instrument.OxfordVRM.lvclass">)
        n127 = call-dynamic "Create Instrument SMO.vi"("error in (no error)"=w357, "Debug Mode? [F]"="Debug Mode", "Configuration Window? [T]"=w359, "Instrument in"=w361) -> ("error out"=w356:errorcluster, "Instrument out"=w358:refnum<class "Instrument.OxfordVRM.lvclass">)  [unwired: 6 in]
        n128 = Bundle By Name(cluster=w362, "Instrument.OxfordVRM"=w358) -> (w363:T4)
        n129 = call <vilib>:"Add State(s) to Queue__jki_lib_state_machine.vi"("State(s) in (\"\")"=w366) -> ("States Out"=w365:string)  [unwired: 14 in]
      }
      frame "SMO: Start Instrument" {
        # "Do not put any code in this frame.\n(It is a separator no-op. You can make a copy of this frame to create a new Macro frame)"
        n130 = Unbundle By Name(w371) -> ("Instrument.OxfordVRM"=w372:refnum<class "Instrument.OxfordVRM.lvclass">)
        n131 = call <vilib>:"Start.vi"("error in (no error)"=w369, "SMO"=w372) -> ("error out"=w368:errorcluster, "SMO out"=w367:refnum<class "Instrument.OxfordVRM.lvclass">)  [unwired: 8 in]
        n132 = Bundle By Name(cluster=w371, "Instrument.OxfordVRM"=w367) -> (w370:T4)
        n133 = call <vilib>:"Add State(s) to Queue__jki_lib_state_machine.vi"("State(s) in (\"\")"=w375) -> ("States Out"=w374:string)  [unwired: 14 in]
      }
      frame "SMO: Stop Instrument" {
        # "Do not put any code in this frame.\n(It is a separator no-op. You can make a copy of this frame to create a new Macro frame)"
        n134 = Unbundle By Name(w383) -> ("Instrument.OxfordVRM"=w381:refnum<class "Instrument.OxfordVRM.lvclass">)
        n135 = call <vilib>:"GetState.vi"("error in (no error)"=w378, "SMO"=w381) -> ("error out"=w377:errorcluster, "SMO State"=w380:T1, "SMO out"=w376:refnum<class "Instrument.OxfordVRM.lvclass">)  [unwired: 7 in]
        n136 = call <vilib>:"Clear Errors.vi"("error in (no error)"=w377) -> ("error out"=w379:errorcluster)  [unwired: 5 in, 1 out]
        n137 = case shown="\"Created\", \"Started\"" w380 {
          tunnel: [w387 w390] -> w382
          tunnel: w379 -> [w387 w389]
          tunnel: w376 -> [_ w388]
          frame Default {
          }
          frame "Created", "Started" {
            n138 = call <vilib>:"Stop.vi"("error in (no error)"=w389, "SMO"=w388) -> ("error out"=w390:errorcluster)  [unwired: 8 in, 1 out]
          }
        }
        n139 = call <vilib>:"Add State(s) to Queue__jki_lib_state_machine.vi"("State(s) in (\"\")"=w386) -> ("States Out"=w385:string)  [unwired: 14 in]
      }
      frame "SMO: Destroy Instrument" {
        # "Do not put any code in this frame.\n(It is a separator no-op. You can make a copy of this frame to create a new Macro frame)"
        n140 = Unbundle By Name(w398) -> ("Instrument.OxfordVRM"=w396:refnum<class "Instrument.OxfordVRM.lvclass">)
        n141 = call <vilib>:"GetState.vi"("error in (no error)"=w393, "SMO"=w396) -> ("error out"=w392:errorcluster, "SMO State"=w395:T1, "SMO out"=w391:refnum<class "Instrument.OxfordVRM.lvclass">)  [unwired: 7 in]
        n142 = call <vilib>:"Clear Errors.vi"("error in (no error)"=w392) -> ("error out"=w394:errorcluster)  [unwired: 5 in, 1 out]
        n143 = case shown="\"Stopped\"" w395 {
          tunnel: [w402 w405] -> w397
          tunnel: w394 -> [w402 w404]
          tunnel: w391 -> [_ w403]
          frame Default {
          }
          frame "Stopped" {
            n144 = call <vilib>:"Destroy.vi"("error in (no error)"=w404, "SMO"=w403) -> ("error out"=w405:errorcluster)  [unwired: 9 in]
          }
        }
        n145 = call <vilib>:"Add State(s) to Queue__jki_lib_state_machine.vi"("State(s) in (\"\")"=w401) -> ("States Out"=w400:string)  [unwired: 14 in]
      }
      frame "SMO: Create Instrument UI" {
        # "Do not put any code in this frame.\n(It is a separator no-op. You can make a copy of this frame to create a new Macro frame)"
        n146 = Unbundle By Name(w412) -> ("Instrument.OxfordVRM UI"=w410:refnum<class "Instrument.OxfordVRM UI.lvclass">, "Instrument.OxfordVRM"=w406:refnum<class "Instrument.OxfordVRM.lvclass">)
        n147 = call <userlib>:"Create UI.vi"("error in (no error)"=w408, "Instrument in"=w406, "Instrument UI"=w410) -> ("error out"=w407:errorcluster, "Instrument UI out"=w409:refnum<class "Instrument.OxfordVRM UI.lvclass">)  [unwired: 7 in]
        n148 = Bundle By Name(cluster=w412, "Instrument.OxfordVRM UI"=w409) -> (w411:T4)
        n149 = call <vilib>:"Add State(s) to Queue__jki_lib_state_machine.vi"("State(s) in (\"\")"=w415) -> ("States Out"=w414:string)  [unwired: 14 in]
      }
      frame "SMO: Start Instrument UI" {
        # "Do not put any code in this frame.\n(It is a separator no-op. You can make a copy of this frame to create a new Macro frame)"
        n150 = Unbundle By Name(w419) -> ("Instrument.OxfordVRM UI"=w418:refnum<class "Instrument.OxfordVRM UI.lvclass">)
        n151 = call <vilib>:"Start.vi"("error in (no error)"=w417, "SMO"=w418) -> ("error out"=w416:errorcluster)  [unwired: 8 in, 1 out]
        n152 = call <vilib>:"Add State(s) to Queue__jki_lib_state_machine.vi"("State(s) in (\"\")"=w422) -> ("States Out"=w421:string)  [unwired: 14 in]
      }
      frame "SMO: Show Instrument UI" {
        # "Do not put any code in this frame.\n(It is a separator no-op. You can make a copy of this frame to create a new Macro frame)"
        n153 = Unbundle By Name(w430) -> ("Instrument.OxfordVRM UI"=w428:refnum<class "Instrument.OxfordVRM UI.lvclass">)
        n154 = call <vilib>:"GetState.vi"("error in (no error)"=w426, "SMO"=w428) -> ("error out"=w424:errorcluster, "SMO State"=w423:T1, "SMO out"=w427:refnum<class "Instrument.OxfordVRM UI.lvclass">)  [unwired: 7 in]
        n155 = call <vilib>:"Clear Errors.vi"("error in (no error)"=w424) -> ("error out"=w425:errorcluster)  [unwired: 5 in, 1 out]
        n156 = case shown="\"Started\"" w423 {
          tunnel: [w434 w437] -> w429
          tunnel: w427 -> [_ w436]
          tunnel: w425 -> [w434 w435]
          frame Default {
          }
          frame "Started" {
            n157 = call <vilib>:"Show.vi"("error in (no error)"=w435, "SMO.UI"=w436) -> ("error out"=w437:errorcluster)  [unwired: 8 in, 1 out]
          }
        }
        n158 = call <vilib>:"Add State(s) to Queue__jki_lib_state_machine.vi"("State(s) in (\"\")"=w433) -> ("States Out"=w432:string)  [unwired: 14 in]
      }
      frame "SMO: Hide Instrument UI" {
        # "Do not put any code in this frame.\n(It is a separator no-op. You can make a copy of this frame to create a new Macro frame)"
        n159 = Unbundle By Name(w445) -> ("Instrument.OxfordVRM UI"=w443:refnum<class "Instrument.OxfordVRM UI.lvclass">)
        n160 = call <vilib>:"GetState.vi"("error in (no error)"=w441, "SMO"=w443) -> ("error out"=w439:errorcluster, "SMO State"=w438:T1, "SMO out"=w442:refnum<class "Instrument.OxfordVRM UI.lvclass">)  [unwired: 7 in]
        n161 = call <vilib>:"Clear Errors.vi"("error in (no error)"=w439) -> ("error out"=w440:errorcluster)  [unwired: 5 in, 1 out]
        n162 = case shown="\"Started\"" w438 {
          tunnel: [w449 w452] -> w444
          tunnel: w442 -> [_ w451]
          tunnel: w440 -> [w449 w450]
          frame Default {
          }
          frame "Started" {
            n163 = call <vilib>:"Hide.vi"("error in (no error)"=w450, "SMO.UI"=w451) -> ("error out"=w452:errorcluster)  [unwired: 8 in, 1 out]
          }
        }
        n164 = call <vilib>:"Add State(s) to Queue__jki_lib_state_machine.vi"("State(s) in (\"\")"=w448) -> ("States Out"=w447:string)  [unwired: 14 in]
      }
      frame "SMO: Stop Instrument UI" {
        # "Do not put any code in this frame.\n(It is a separator no-op. You can make a copy of this frame to create a new Macro frame)"
        n165 = Unbundle By Name(w459) -> ("Instrument.OxfordVRM UI"=w454:refnum<class "Instrument.OxfordVRM UI.lvclass">)
        n166 = call <vilib>:"GetState.vi"("error in (no error)"=w458, "SMO"=w454) -> ("error out"=w457:errorcluster, "SMO State"=w455:T1, "SMO out"=w453:refnum<class "Instrument.OxfordVRM UI.lvclass">)  [unwired: 7 in]
        n167 = call <vilib>:"Clear Errors.vi"("error in (no error)"=w457) -> ("error out"=w456:errorcluster)  [unwired: 5 in, 1 out]
        n168 = case shown="\"Created\", \"Started\"" w455 {
          tunnel: [w464 w467] -> w460
          tunnel: w453 -> [_ w466]
          tunnel: w456 -> [w464 w465]
          frame Default {
          }
          frame "Created", "Started" {
            n169 = call <vilib>:"Stop.vi"("error in (no error)"=w465, "SMO"=w466) -> ("error out"=w467:errorcluster)  [unwired: 8 in, 1 out]
          }
        }
        n170 = call <vilib>:"Add State(s) to Queue__jki_lib_state_machine.vi"("State(s) in (\"\")"=w463) -> ("States Out"=w462:string)  [unwired: 14 in]
      }
      frame "SMO: Destroy Instrument UI" {
        # "Do not put any code in this frame.\n(It is a separator no-op. You can make a copy of this frame to create a new Macro frame)"
        n171 = Unbundle By Name(w474) -> ("Instrument.OxfordVRM UI"=w473:refnum<class "Instrument.OxfordVRM UI.lvclass">)
        n172 = call <vilib>:"GetState.vi"("error in (no error)"=w471, "SMO"=w473) -> ("error out"=w470:errorcluster, "SMO State"=w468:T1, "SMO out"=w472:refnum<class "Instrument.OxfordVRM UI.lvclass">)  [unwired: 7 in]
        n173 = call <vilib>:"Clear Errors.vi"("error in (no error)"=w470) -> ("error out"=w469:errorcluster)  [unwired: 5 in, 1 out]
        n174 = case shown="\"Stopped\"" w468 {
          tunnel: w469 -> [w479 w482]
          tunnel: [w479 w481] -> w475
          tunnel: w472 -> [_ w480]
          frame Default {
          }
          frame "Stopped" {
            n175 = call <vilib>:"Destroy.vi"("error in (no error)"=w482, "SMO"=w480) -> ("error out"=w481:errorcluster)  [unwired: 9 in]
          }
        }
        n176 = call <vilib>:"Add State(s) to Queue__jki_lib_state_machine.vi"("State(s) in (\"\")"=w478) -> ("States Out"=w477:string)  [unwired: 14 in]
      }
      frame "---------- Splash ----------" {
        # "Template Separator\n(You can make a copy of, or modify, this frame)"
        n177 = call <vilib>:"Add State(s) to Queue__jki_lib_state_machine.vi"("State(s) in (\"\")"=w487) -> ("States Out"=w486:string)  [unwired: 14 in]
      }
      frame "Splash: Set Status" {
        # "Your code here.\n(You can make a copy of, or modify, this frame)"
        n178 = property on="Splash Status" class="Str"(error in=w490, "Value"=w491) -> (error out=w489:errorcluster)  [unwired: 1 in, 1 out]
        n179 = call <vilib>:"Add State(s) to Queue__jki_lib_state_machine.vi"("State(s) in (\"\")"=w494) -> ("States Out"=w493:string)  [unwired: 14 in]
      }
      frame "Splash: 2" {
        # "Your code here.\n(You can make a copy of, or modify, this frame)"
        n180 = call <vilib>:"Add State(s) to Queue__jki_lib_state_machine.vi"("State(s) in (\"\")"=w499) -> ("States Out"=w498:string)  [unwired: 14 in]
      }
    }
  }
  "error out" <- w1
